vi "PASCO_PID.vi"(0 "Delta":dbl(slide) scale=-1.0..1.0, 9 "Integral Reset":bool, 12 "P Gain":dbl=1.0, 13 "I Gain":dbl, 14 "D Gain":dbl) -> (4 "HarvOutElev":dbl)   [LabVIEW 2012]
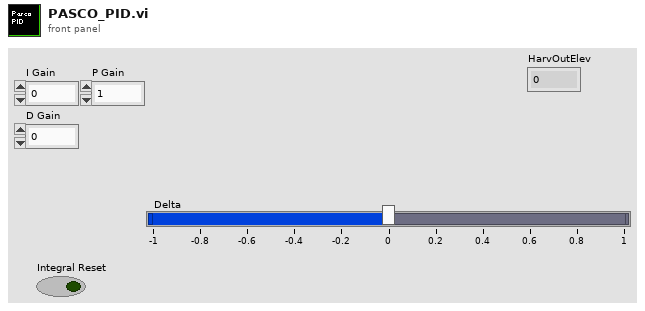
[diagram p1: front panel]
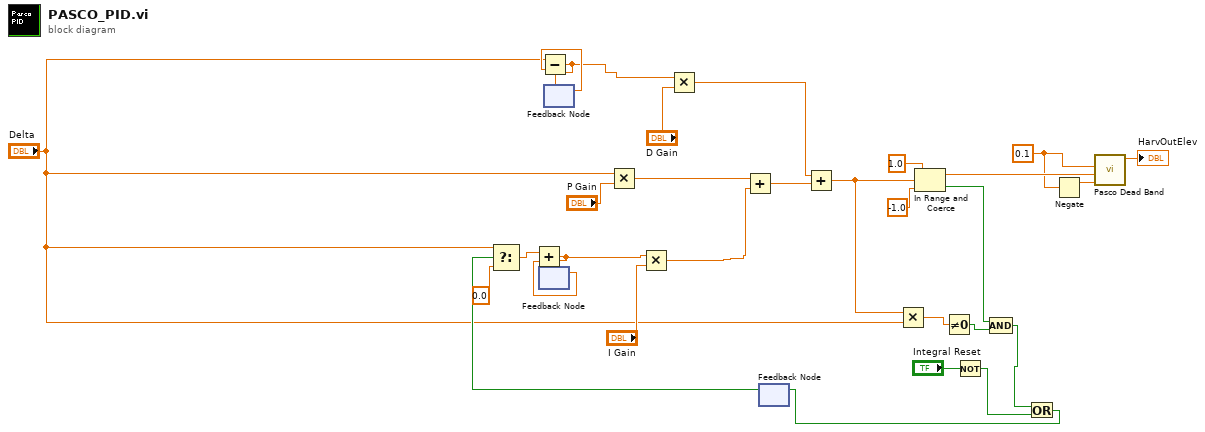
[diagram p0: block diagram]
diagram:
  w15 = 0.1 ("upper limit")
  n1 = feedback #1() -> (w3:dbl)  [unwired: 1 in]
  n2 = feedback #2() -> (w26:dbl)  [unwired: 1 in]
  n3 = Subtract(x="Delta", y=w26) -> (x-y=w4:dbl)
  n4 = feedback-in #2(w4) -> ()
  n5 = Multiply(x="Delta", y="P Gain") -> (x*y=w12:dbl)
  n6 = Multiply(x=w4, y="D Gain") -> (x*y=w5:dbl)
  n7 = feedback #3() -> (w14:bool)  [unwired: 1 in]
  n8 = Select(t="Delta", s=w14, f=0.0) -> (s? t:f=w20:dbl)
  n9 = Add(x=w20, y=w3) -> (x+y=w2:dbl)
  n10 = feedback-in #1(w2) -> ()
  n11 = Multiply(x=w2, y="I Gain") -> (x*y=w6:dbl)
  n12 = Add(x=w12, y=w6) -> (x+y=w19:dbl)
  n13 = Add(x=w5, y=w19) -> (x+y=w18:dbl)
  n14 = Multiply(x=w18, y="Delta") -> (x*y=w24:dbl)
  n15 = In Range and Coerce(upper limit=1.0, x=w18, lower limit=-1.0) -> (coerced(x)=w17:dbl, In Range?=w22:bool)
  n16 = Not Equal To 0?(x=w24) -> (x != 0?=w23:bool)
  n17 = Not(x="Integral Reset") -> (.not. x?=w9:bool)
  n18 = Compound Arithmetic op=AND(w22, w23) -> (w10:bool)
  n19 = Or(x=w10, y=w9) -> (x .or. y?=w8:bool)
  n20 = feedback-in #3(w8) -> ()
  n21 = Negate(x=w15) -> (-x=w16:dbl)
  n22 = call "Pasco Dead Band.vi"("lower limit"=w16, "PWM Power"=w17, "upper limit"=w15) -> ("PWM Power"=→"HarvOutElev":dbl)  [unwired: 7 in, 1 out]
